vi "Word Search.vi"() -> ()   [LabVIEW 2020]
panel:
  in  "Run Example":bool
  out "All Words Found":bool
  out "Execution Time":dbl
  in  "Word List":string[](array[string])=["YELLOW", "ORANGE", "PURPLE", "BLUE", "GREEN", "RED"]
  in  "Word Search Grid":string[][](array[string])=[["R", "B", "L", "U", "E", "W"], ["E", "G", "N", "A", "R", "O"], ["D", "B", "C", "E", "W", "L"], ["L", "L", "D", "K", "V", "L"], ["P", "U", "R", "P", "L", "E"], ["N", "E", "E", "R", "G", "Y"]]
  # "Use this Test Harness VI to time your Word Search solution (and ensure it works correctly)."
  # "Your Solver"
  # "Example Solver"
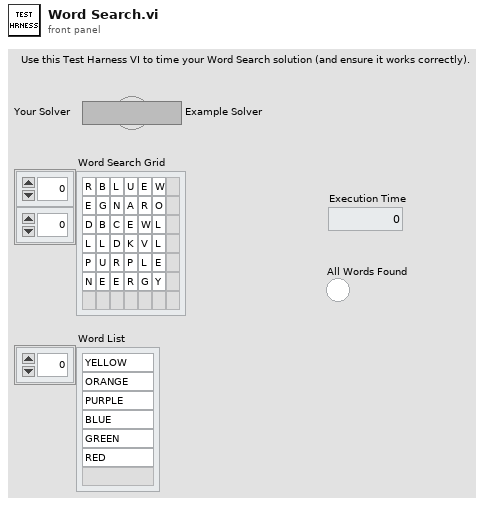
[diagram p1: front panel]
types:
  T1 = typedef "Solutions--map.ctl" = map{string, T2[]}
  T2 = typedef "Letter Index--cluster.ctl" = cluster{"Row":i32, "Column":i32}
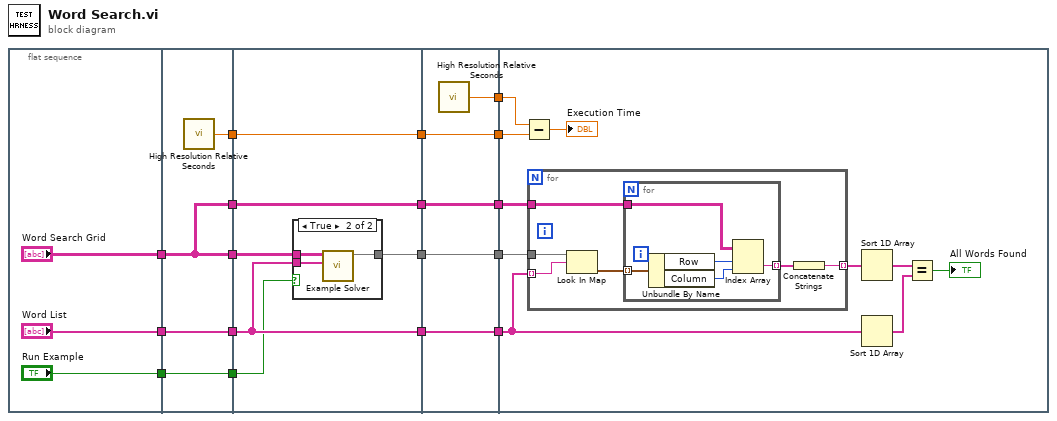
[diagram p0: block diagram]
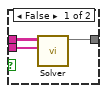
[diagram p2: hidden frame]
diagram:
  n1 = flat-sequence {
    tunnel: ["Word Search Grid"] -> w17
    tunnel: ["Word List"] -> w16
    tunnel: ["Run Example"] -> w1
    tunnel: w17 -> [w22]
    tunnel: w16 -> [w24]
    tunnel: [w24] -> w15
    tunnel: [w22] -> w14
    tunnel: [w23] -> w10
    tunnel: [w22] -> w3
    tunnel: [w21] -> w2
    tunnel: w1 -> [w21]
    tunnel: w15 -> [w27]
    tunnel: w14 -> [w30]
    tunnel: [w29] -> w13
    tunnel: w10 -> [w28]
    tunnel: [w28] -> w9
    tunnel: [w27] -> w6
    tunnel: [w26] -> w4
    tunnel: w3 -> [w26]
    tunnel: w2 -> [w25]
    tunnel: w13 -> [w41]
    tunnel: [w41] -> w12
    tunnel: [w40] -> w11
    tunnel: w9 -> [w39]
    tunnel: [w39] -> w8
    tunnel: [w38] -> w7
    tunnel: w6 -> [w38]
    tunnel: [w37] -> w5
    tunnel: w4 -> [w37]
    tunnel: w12 -> [w48]
    tunnel: w11 -> [w51]
    tunnel: w8 -> [w50]
    tunnel: w7 -> [w45]
    tunnel: w5 -> [w47]
    frame #0 {
    }
    frame #1 {
      n2 = call <vilib>:"High Resolution Relative Seconds.vi"() -> ("relative seconds"=w23:dbl)
    }
    frame #2 {
      n3 = case shown="True" w25 {
        tunnel: w30 -> [w33 w36]
        tunnel: [w31 w35] -> w29
        tunnel: w27 -> [w32 w34]
        frame False {
          n4 = call "Solver.vi"("Word List"=w32, "Word Search Grid"=w33) -> ("Solutions"=w31:T1)  [unwired: 9 in]
        }
        frame True {
          n5 = call "Example Solver.vi"("Word List"=w34, "Word Search Grid"=w36) -> ("Solutions"=w35:T1)  [unwired: 9 in]
        }
      }
    }
    frame #3 {
      n6 = call <vilib>:"High Resolution Relative Seconds.vi"() -> ("relative seconds"=w40:dbl)
    }
    frame #4 {
      n7 = Subtract(x=w51, y=w50) -> (x-y=→"Execution Time":dbl)
      n8 = for {
        tunnel: w45 -> [w56] mode=indexing
        tunnel: w48 -> [w57]
        tunnel: w47 -> [w54]
        tunnel: [w52] -> w46 mode=indexing
        n9 = Look In Map(map=w57, key=w56) -> (value=w55:T2[])  [unwired: 1 in, 1 out]
        n10 = for {
          tunnel: w55 -> [w62] mode=indexing
          tunnel: w54 -> [w60]
          tunnel: [w58] -> w53 mode=indexing
          n11 = Unbundle By Name(w62) -> ("Row"=w61:i32, "Column"=w59:i32)
          n12 = Index Array(array=w60, index (row)=w61, index (col)=w59) -> (element=w58:string)
        }
        n13 = Concatenate Strings(w53) -> (w52:string)
      }
      n14 = Sort 1D Array(array=w46) -> (sorted array=w44:string[])
      n15 = Sort 1D Array(array=w45) -> (sorted array=w43:string[])
      n16 = Equal?(x=w44, y=w43) -> (x = y?=→"All Words Found":bool)
    }
  }
